vi "Can Move From.vi"(10 "Room":string[](array[string]), 11 "Amphipod":string) -> (3 "Can Move From?":bool)   [LabVIEW 2019, in "23.lvlib"]
uses:
  23.lvlib
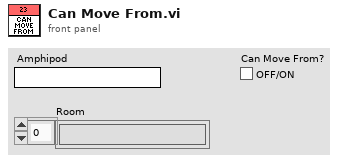
[diagram p1: front panel]
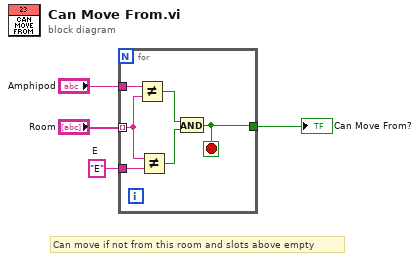
[diagram p0: block diagram]
diagram:
  w4 = "E"  # E
  # "Can move if not from this room and slots above empty"
  n1 = for {
    tunnel: "Room" -> [w9] mode=indexing
    tunnel: "Amphipod" -> [w10]
    tunnel: w4 -> [w8]
    tunnel: [w5] -> w3
    stop <- w5 stop-if-true
    n2 = Not Equal?(x=w10, y=w9) -> (x != y?=w7:bool)
    n3 = Not Equal?(x=w9, y=w8) -> (x != y?=w6:bool)
    n4 = And(x=w7, y=w6) -> (x .and. y?=w5:bool)
  }
  "Can Move From?" <- w3
